vi "Data Bank (2D).vi"(1 "Action":T1(ring), 7 "1D Data in":dbl[](array[numeric]), 11 "n":i32) -> (4 "2D Data out":dbl[][](array[numeric]), 8 "1D Data out":dbl[](array[numeric]), 15 "Nrows":i32)   [LabVIEW 2015]
uses:
  Utility VIs/Array Dimensions (2D).vi
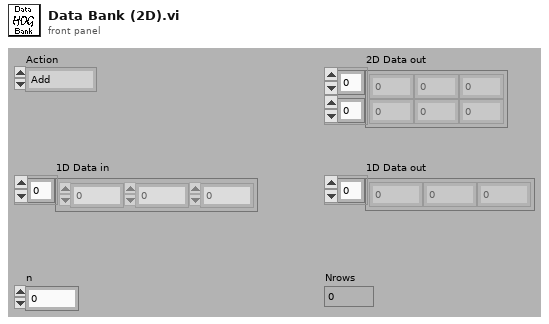
[diagram p1: front panel]
types:
  T1 = enum16{"Add", "Clear", "Read", "Read nth", "Replace nth"}
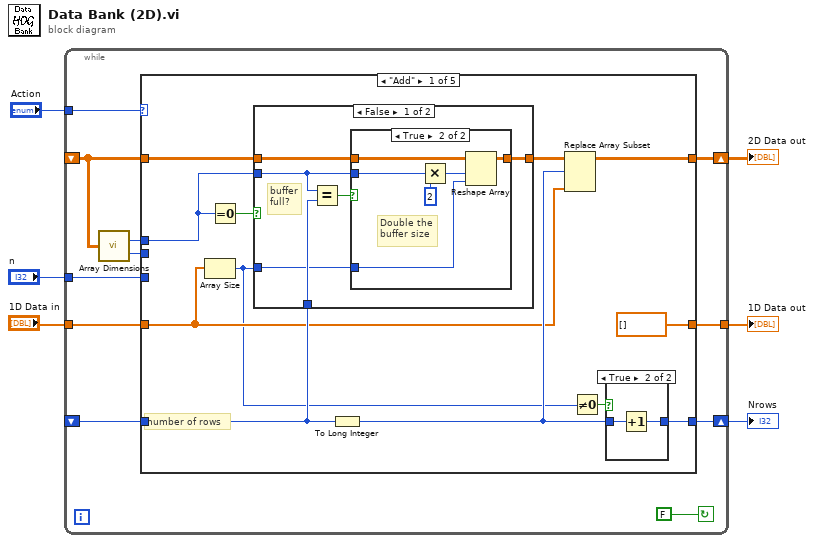
[diagram p0: block diagram]
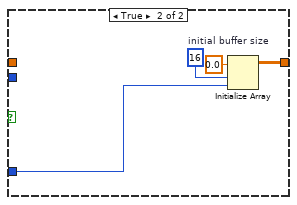
[diagram p4: hidden frame]
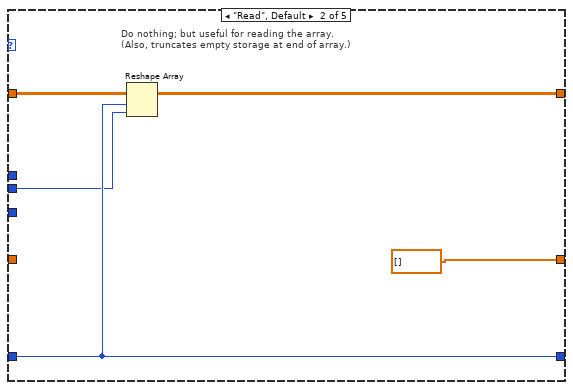
[diagram p5: hidden frame]
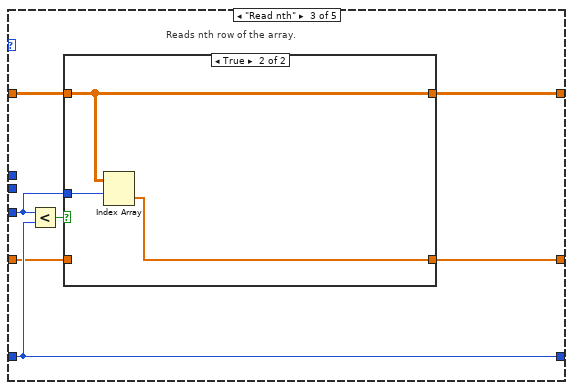
[diagram p6: hidden frame]
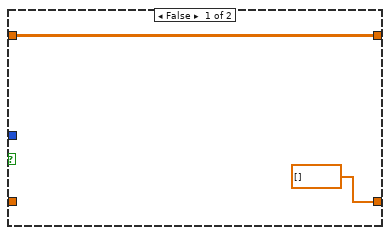
[diagram p7: hidden frame]
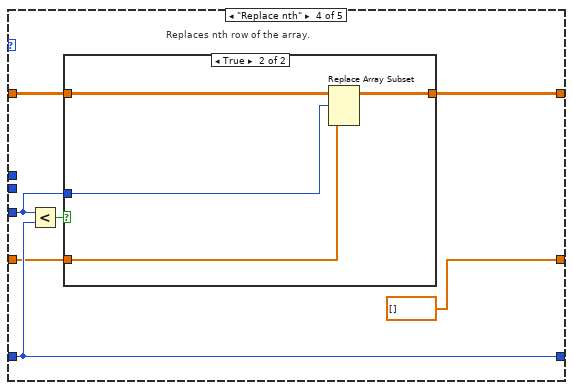
[diagram p8: hidden frame]
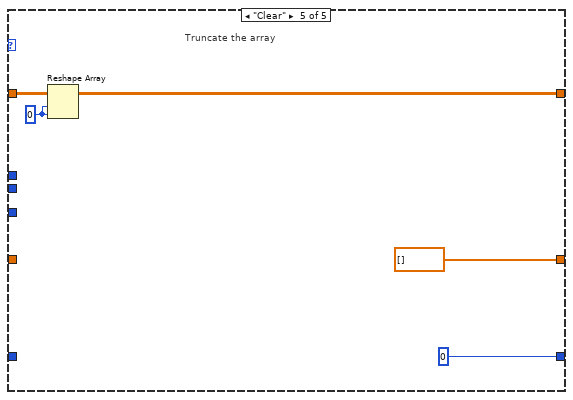
[diagram p10: hidden frame]
diagram:
  n1 = while {
    tunnel: "1D Data in" -> [w13]
    shift-left: _ -> [w15]
    shift-right: [w14] -> w5
    shift-left: _ -> [w9]
    shift-right: [w16] -> w3
    tunnel: "Action" -> [w17]
    tunnel: "n" -> [w11]
    tunnel: [w10] -> w2
    stop <- FALSE continue-if-true
    n2 = call-poly "Array Dimensions.vi"("2D Array"=w9) -> ("# rows"=w8:i32, "# columns"=w7:i32)  [unwired: 13 in]
    n3 = case shown="\"Add\"" w17 {
      tunnel: w9 -> [w27 w53 w59 w71 w83]
      tunnel: [w24 w54 w58 w70 w82] -> w16
      tunnel: w15 -> [w28 w51 w61 w73 _]
      tunnel: [w29 w51 w61 w73 0] -> w14
      tunnel: w13 -> [w22 _ w56 w68 _]
      tunnel: w11 -> [_ _ w57 w69 _]
      tunnel: [dbl[] [] ("2D Data in") dbl[] [] ("2D Data in") w55 dbl[] [] ("2D Data in") dbl[] [] ("2D Data in")] -> w10
      tunnel: w8 -> [w21 _ _ _ _]
      tunnel: w7 -> [_ w50 _ _ _]
      frame "Add" {
        # "number of rows"
        n4 = Array Size(array=w22) -> (size(s)=w18:i32)
        n5 = Equal To 0?(x=w21) -> (x = 0?=w20:bool)
        n6 = case shown="False" w20 {
          tunnel: w28 -> [w37 _]
          tunnel: w27 -> [w36 _]
          tunnel: [w35 w47] -> w25
          tunnel: w18 -> [w34 w48]
          tunnel: w21 -> [w33 _]
          frame False {
            # "buffer\nfull?"
            n7 = Equal?(x=w33, y=w37) -> (x = y?=w38:bool)
            n8 = case shown="True" w38 {
              tunnel: w36 -> [w39 w45]
              tunnel: [w39 w44] -> w35
              tunnel: w33 -> [_ w42]
              tunnel: w34 -> [_ w43]
              frame False {
              }
              frame True {
                # "Double the\nbuffer size"
                n9 = Multiply(x=w42, y=2) -> (x*y=w40:i32)
                n10 = Reshape Array(w45, w40, w43) -> (w44:dbl[][])
              }
            }
          }
          frame True {
            w49 = 16  # initial buffer size
            n11 = Initialize Array(0.0 ("element"), w49, w48) -> (w47:dbl[][])
          }
        }
        n12 = To Long Integer(number=w28) -> (32bit integer=w23:i32)
        n13 = Replace Array Subset(array=w25, new element=w22, index (row)=w23) -> (w24:dbl[][])  [unwired: 1 in]
        n14 = Not Equal To 0?(x=w18) -> (x != 0?=w19:bool)
        n15 = case shown="True" w19 {
          tunnel: [w30 w32] -> w29
          tunnel: w23 -> [w30 w31]
          frame False {
          }
          frame True {
            n16 = Increment(x=w31) -> (x+1=w32:i32)
          }
        }
      }
      frame "Read", Default {
        # "Do nothing; but useful for reading the array.\n(Also, truncates empty storage at end of array.)"
        n17 = Reshape Array(w53, w51, w50) -> (w54:dbl[][])
      }
      frame "Read nth" {
        # "Reads nth row of the array."
        n18 = Less?(x=w57, y=w61) -> (x < y?=w60:bool)
        n19 = case shown="True" w60 {
          tunnel: w59 -> [w63 w65]
          tunnel: [w63 w65] -> w58
          tunnel: w57 -> [_ w64]
          tunnel: w56 -> [_ _]
          tunnel: [dbl[] [] ("Modified 2D Array") w66] -> w55
          frame False {
          }
          frame True {
            n20 = Index Array(array=w65, index (row)=w64) -> (element=w66:dbl[])  [unwired: 1 in]
          }
        }
      }
      frame "Replace nth" {
        # "Replaces nth row of the array."
        n21 = Less?(x=w69, y=w73) -> (x < y?=w72:bool)
        n22 = case shown="True" w72 {
          tunnel: w71 -> [w74 w78]
          tunnel: [w74 w77] -> w70
          tunnel: w69 -> [_ w76]
          tunnel: w68 -> [_ w75]
          frame False {
          }
          frame True {
            n23 = Replace Array Subset(array=w78, new element=w75, index (row)=w76) -> (w77:dbl[][])  [unwired: 1 in]
          }
        }
      }
      frame "Clear" {
        w80 = 0
        # "Truncate the array"
        n24 = Reshape Array(w83, w80, w80) -> (w82:dbl[][])
      }
    }
  }
  "Nrows" <- w5
  "2D Data out" <- w3
  "1D Data out" <- w2
